vi "rotate_and_reflect_point.vi"(9 "Point":cluster{"X":sgl, "Y":sgl} {"Y" format="%.2f"; "X" format="%.2f"}, 10 "reflect about the x axis?":bool, 11 "rotation angle (radians)":sgl) -> (1 "transformed point":cluster{"X":sgl, "Y":sgl} {"Y" format="%.2f"; "X" format="%.2f"})   [LabVIEW 2019]
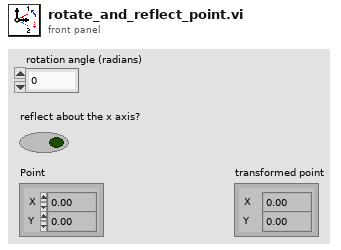
[diagram p1: front panel]
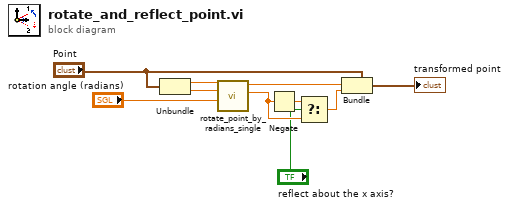
[diagram p0: block diagram]
diagram:
  n1 = Unbundle("Point") -> ("X"=w10:sgl, "Y"=w9:sgl)
  n2 = call "rotate_point_by_radians_single.vi"("theta"="rotation angle (radians)", "y"=w9, "x"=w10) -> ("y out"=w7:sgl, "x out"=w5:sgl)  [unwired: 7 in]
  n3 = Negate(x=w7) -> (-x=w8:sgl)
  n4 = Select(t=w8, s="reflect about the x axis?", f=w7) -> (s? t:f=w6:sgl)
  n5 = Bundle(cluster="Point", "X"=w5, "Y"=w6) -> (→"transformed point":cluster{"X":sgl, "Y":sgl})
